vi "ph_case.vi"() -> ()   [LabVIEW 2011]
panel:
  out "number":u32
  out "appended array":bool[](array[boolean])
  out "x > 0? 6":bool
  out "x > 0? 5":bool
  out "x > 0? 4":bool
  out "x > 0? 3":bool
  out "x > 0? 2":bool
  out "x > 0?":bool
  in  "x 6":dbl
  in  "x 5":dbl
  in  "x 4":dbl
  in  "x 3":dbl
  in  "x 2":dbl
  in  "x":dbl
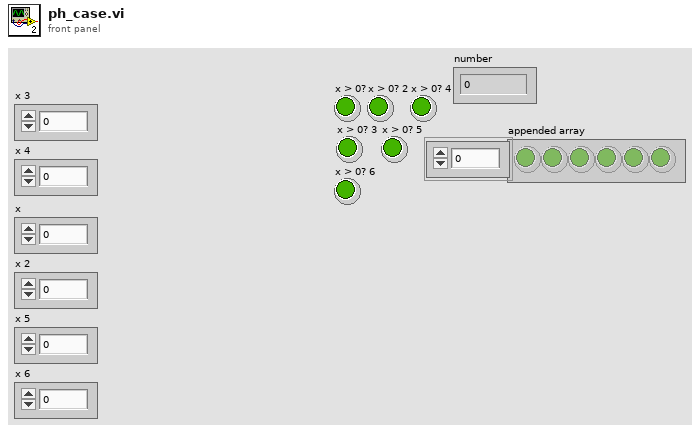
[diagram p1: front panel]
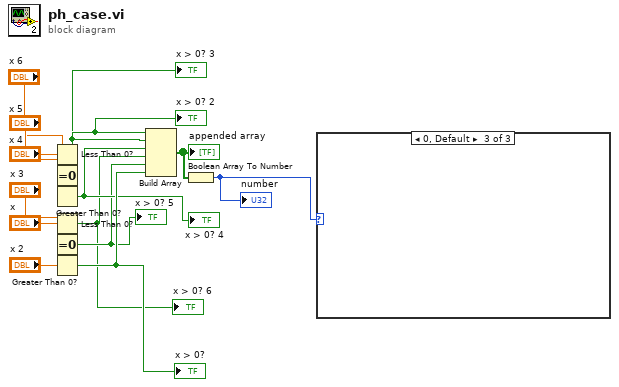
[diagram p0: block diagram]
diagram:
  n1 = Less Than 0?(x="x 4") -> (x < 0?=w5:bool)
  "x > 0? 2" <- w5
  n2 = Equal To 0?(x="x 6") -> (x = 0?=w4:bool)
  "x > 0? 3" <- w4
  n3 = Greater Than 0?(x="x 5") -> (x > 0?=w3:bool)
  "x > 0? 4" <- w3
  n4 = Less Than 0?(x="x") -> (x < 0?=w1:bool)
  "x > 0? 6" <- w1
  n5 = Equal To 0?(x="x 3") -> (x = 0?=w2:bool)
  "x > 0? 5" <- w2
  n6 = Greater Than 0?(x="x 2") -> (x > 0?=w13:bool)
  "x > 0?" <- w13
  n7 = Build Array(w5, w4, w3, w1, w2, w13) -> (w12:bool[])
  "appended array" <- w12
  n8 = Boolean Array To Number(Boolean array=w12) -> (number=w14:u32)
  "number" <- w14
  n9 = case shown="0, Default" w14 {
    frame 1 {
    }
    frame 36 {
    }
    frame 0, Default {
    }
  }
